vi "Retrieve Element.vi"(7 "Endpoint element key":string, 8 "error in (no error)":errorcluster, 10 "Token element":T1, 11 "OAuthAccessToken in":refnum<class "OAuthAccessToken.lvclass">) -> (0 "error out":errorcluster, 1 "Value":string, 2 "Key":string, 3 "OAuthAccessToken out":refnum<class "OAuthAccessToken.lvclass">)   [LabVIEW 2013, in "OAuthAccessToken.lvclass"]
uses:
  OAuthAccessToken.lvclass
  OAuth2 Token Element -- enum.ctl
  OAuthAccessToken.lvclass/OAuthAccessToken.ctl
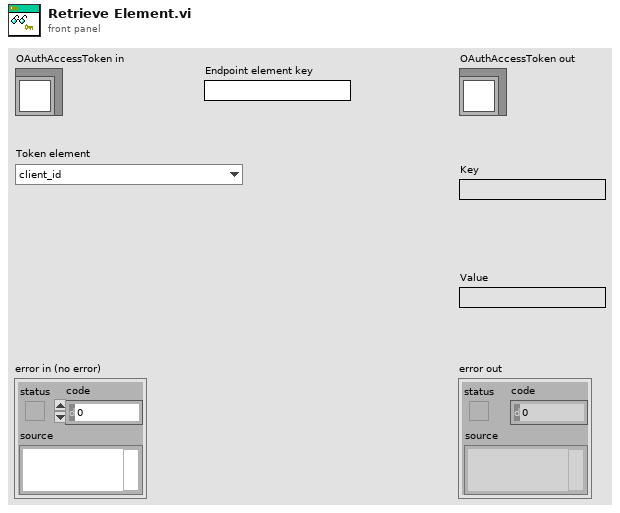
[diagram p1: front panel]
types:
  T1 = typedef "OAuthAccessToken.lvclass/OAuth2 Token Element -- enum.ctl" = enum16{"client_id", "client_secret", "response_type", "scope", "redirect_uri", "error", "error_description", "error_uri", "grant_type", "code", "access_token", "token_type", "expires_in", "username", "password", "refresh_token", "code_challenge", "code_verifier", "code_challenge_method", "endpoint element"}
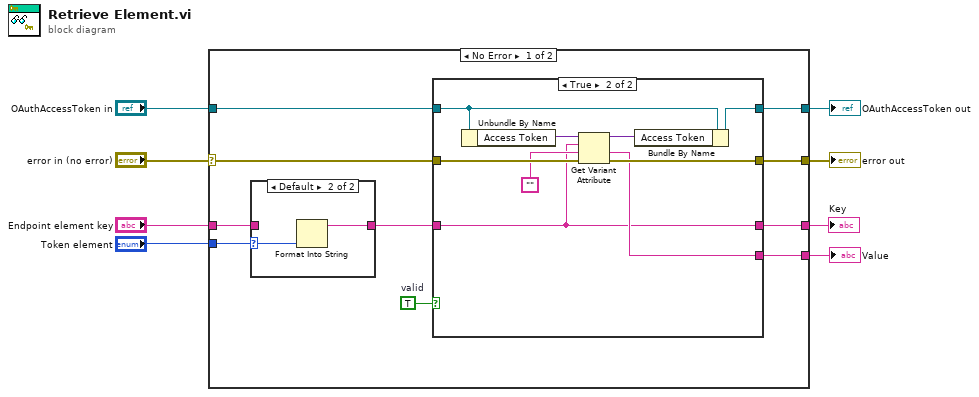
[diagram p0: block diagram]
diagram:
  n1 = case shown="No Error" "error in (no error)" {
    selector: "error in (no error)" -> [w14 w35]
    tunnel: [w13 w35] -> w7
    tunnel: [w17 w34] -> w5
    tunnel: "OAuthAccessToken in" -> [w18 w34]
    tunnel: "Token element" -> [w12 _]
    tunnel: "Endpoint element key" -> [w11 _]
    tunnel: [w10 _] -> w2
    tunnel: [w9 _] -> w1
    frame No Error {
      w15 = TRUE  # valid
      n2 = case shown="Default" w12 {
        selector: w12 -> [_ w20]
        tunnel: [w19 w21] -> w16
        tunnel: w11 -> [w19 _]
        frame "endpoint element" {
        }
        frame Default {
          n3 = Format Into String(w20) -> (resulting string=w21:string)  [unwired: 3 in, 1 out]
        }
      }
      n4 = case shown="True" w15 {
        tunnel: w18 -> [w24 w33]
        tunnel: [w24 w32] -> w17
        tunnel: w16 -> [w22 w25]
        tunnel: w14 -> [w23 w29]
        tunnel: [w23 w28] -> w13
        tunnel: [_ w27] -> w10
        tunnel: [w22 w25] -> w9
        frame False {
        }
        frame True {
          n5 = Unbundle By Name(w33) -> ("Access Token"=w31:variant)
          n6 = Get Variant Attribute(Variant=w31, name=w25, default value (empty Variant)="", error in=w29) -> (duplicate Variant=w30:variant, value=w27:string, error out=w28:errorcluster)  [unwired: 1 out]
          n7 = Bundle By Name(cluster=w33, "Access Token"=w30) -> (w32:refnum<class "OAuthAccessToken.lvclass">)
        }
      }
    }
    frame Error {
    }
  }
  "error out" <- w7
  "OAuthAccessToken out" <- w5
  "Value" <- w2
  "Key" <- w1
